vi "getCodecType.vi"(8 "error in (no error)":errorcluster, 11 "VideoFile in":refnum<class "VideoFile.lvclass">) -> (0 "error out":errorcluster, 2 "codecType":string, 3 "VideoFile out":refnum<class "VideoFile.lvclass">)   [LabVIEW 2017, in "VideoFile.lvclass"]
uses:
  VideoFile.lvclass
  VideoFile.lvclass/VideoFile.ctl
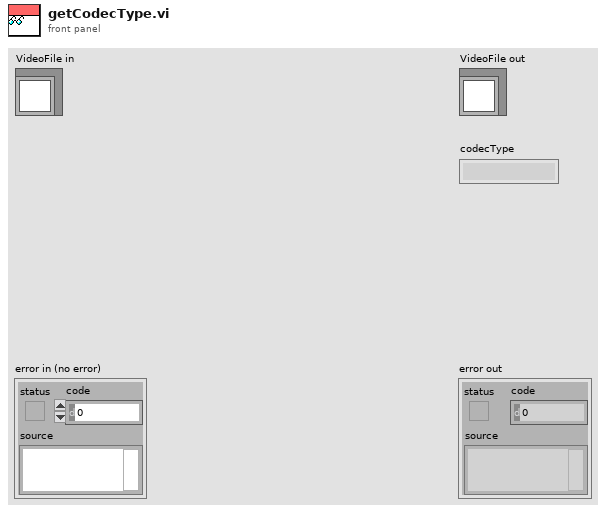
[diagram p1: front panel]
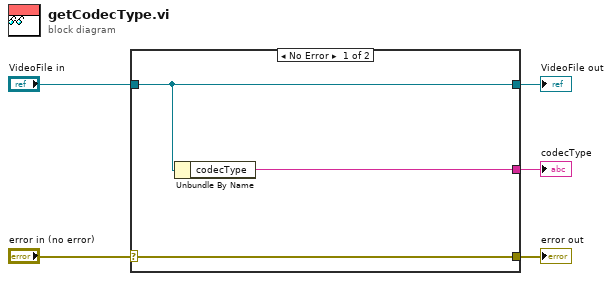
[diagram p0: block diagram]
diagram:
  n1 = case shown="No Error" "error in (no error)" {
    selector: "error in (no error)" -> [w8 w9]
    tunnel: [w8 w9] -> w4
    tunnel: [w7 w10] -> w2
    tunnel: "VideoFile in" -> [w7 w10]
    tunnel: [w6 _] -> w1
    frame No Error {
      n2 = Unbundle By Name(w7) -> ("codecType"=w6:string)
    }
    frame Error {
    }
  }
  "error out" <- w4
  "VideoFile out" <- w2
  "codecType" <- w1
